vi "Process_Arduino_DataPacket.vi"(11 "Data Packet":string) -> (0 "error out":errorcluster, 1 "Sensor Packets Returned":i32, 2 "Sensor Readings (Signed)":i16[](array[numeric]), 3 "Time":u32)   [LabVIEW 2016]
panel:
  out "raw byte array":u8[](array[numeric])
  out "Time Packet":string
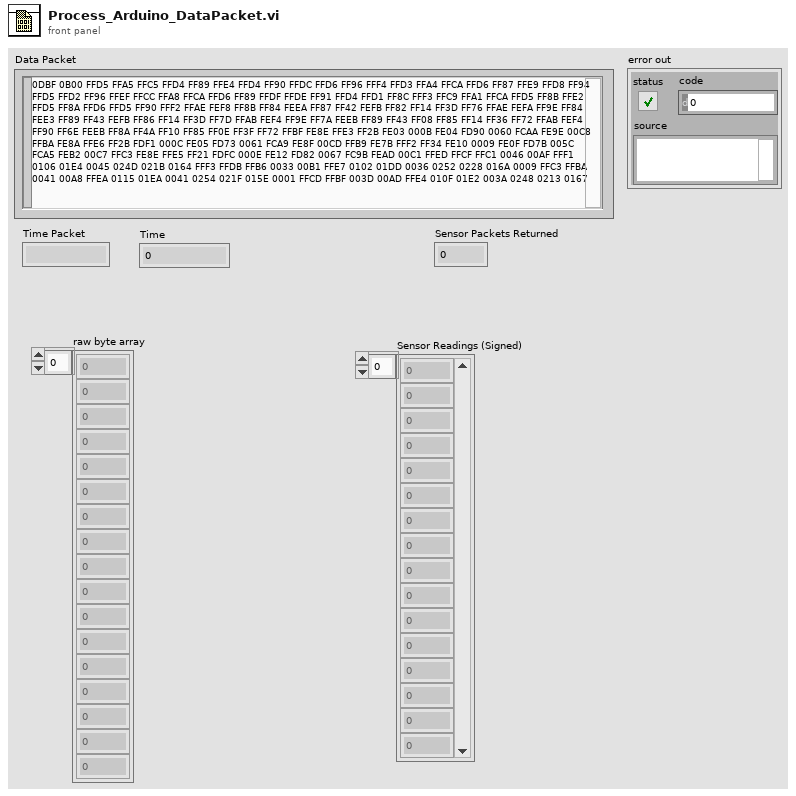
[diagram p1: front panel]
types:
  T1 = enum16{"big-endian, network order", "native, host order", "little-endian"}
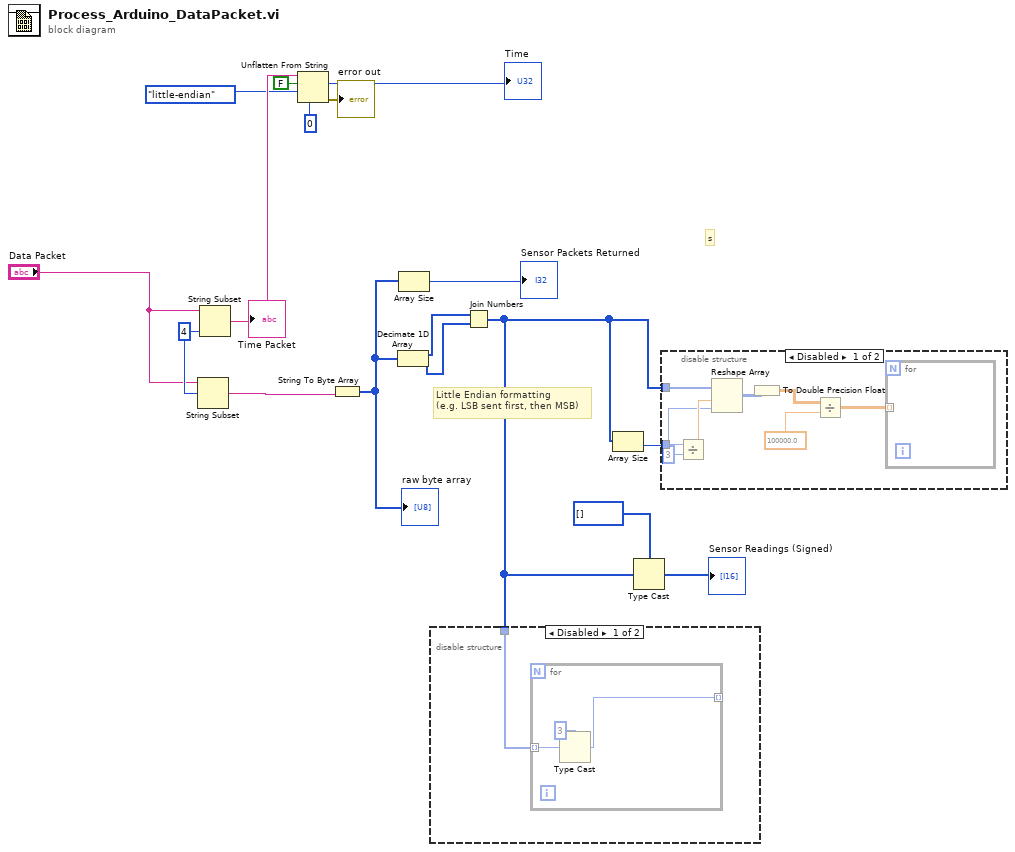
[diagram p0: block diagram]
diagram:
  w17 = 4 ("length (rest)")
  # "s"
  # "Little Endian formatting\n(e.g. LSB sent first, then MSB)"
  n1 = String Subset(string="Data Packet", offset (0)=w17) -> (substring=w13:string)  [unwired: 1 in]
  n2 = String Subset(string="Data Packet", length (rest)=w17) -> (substring=w16:string)  [unwired: 1 in]
  "Time Packet" <- w16
  n3 = Unflatten From String(type=u32 0 ("default (0 U32)"), binary string=w16, data includes array or string size? (T)=FALSE, byte order (0:big-endian, network order)=T1."little-endian") -> (value=→"Time":u32, error out=→"error out":errorcluster)  [unwired: 1 in, 1 out]
  n4 = String To Byte Array(string=w13) -> (unsigned byte array=w12:u8[])
  "raw byte array" <- w12
  n5 = Decimate 1D Array(w12) -> (w8:u8[], w7:u8[])
  n6 = Array Size(array=w12) -> (size(s)=→"Sensor Packets Returned":i32)
  n7 = Join Numbers(hi=w8, lo=w7) -> ((hi.lo)=w4:u16[])
  n8 = disable-structure shown="Disabled" {
    disable-tunnel: w4 -> [w18 _]
    frame Disabled {
      n9 = for {
        tunnel: w18 -> [w21] mode=indexing
        tunnel: [w19] -> _ mode=indexing
        n10 = Type Cast(type=i16 3 ("y"), x=w21) -> (*(type *) &x=w19:i16)
      }
    }
    frame Enabled {
    }
  }
  n11 = Array Size(array=w4) -> (size(s)=w6:i32)
  n12 = Type Cast(type=i16[] [], x=w4) -> (*(type *) &x=→"Sensor Readings (Signed)":i16[])
  n13 = disable-structure shown="Disabled" {
    disable-tunnel: w6 -> [w29 _]
    disable-tunnel: w4 -> [w22 _]
    frame Disabled {
      w27 = 3 ("y")
      n14 = Divide(x=w29, y=w27) -> (x/y=w28:dbl)
      n15 = Reshape Array(w22, w28, w27) -> (w26:u16[][])
      n16 = To Double Precision Float(number=w26) -> (double precision float=w24:dbl[][])
      n17 = Divide(x=w24, y=100000.0) -> (x/y=w23:dbl[][])
      n18 = for {
        tunnel: w23 -> [_] mode=indexing
      }
    }
    frame Enabled {
    }
  }
